vi "Create Link.vi"(8 "Error In":errorcluster, 9 "Remote Link Path":string, 10 "Remote Source Path":string, 11 "SFTP In":refnum<class "SFTP.lvclass">) -> (0 "Error Out":errorcluster, 3 "SFTP Out":refnum<class "SFTP.lvclass">)   [LabVIEW 2018, in "Toolkit.lvlib" / "SFTP.lvclass"]
uses:
  SFTP.lvclass
  SFTP.lvclass/SFTP.ctl
  Session/Session.lvclass/Session.ctl
  SSH/SSH.lvclass/SSH.ctl
  Toolkit.lvlib
  Session/Session.lvclass
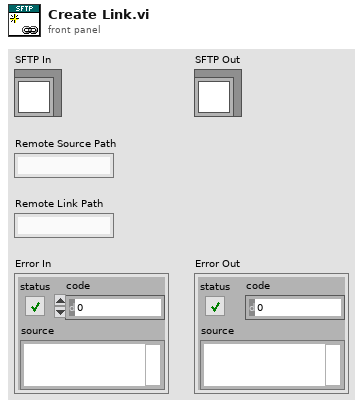
[diagram p1: front panel]
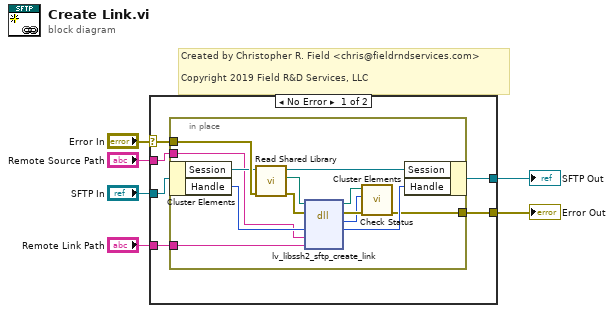
[diagram p0: block diagram]
diagram:
  # "Created by Christopher R. Field <chris@fieldrndservices.com>\n\nCopyright 2019 Field R&D Services, LLC"
  n1 = case shown="No Error" "Error In" {
    selector: "Error In" -> [w12 w27]
    tunnel: [w11 w27] -> w5
    tunnel: "SFTP In" -> [w10 w26]
    tunnel: [w9 w26] -> w3
    tunnel: "Remote Source Path" -> [w8 _]
    tunnel: "Remote Link Path" -> [w7 _]
    frame No Error {
      n2 = in-place {
        in-place-border: w12 -> [w20]
        in-place-border: [w21] -> w11
        in-place-border: w8 -> [w14]
        in-place-border: w7 -> [w13]
        n3 = in-place-cluster #1(w10) -> ("Session"=w19:refnum<class "Session.lvclass">, "Handle"=w15:u64)
        n4 = call "Read Shared Library.vi"("Error In"=w20, "Session In"=w19) -> ("Erorr Out"=w17:errorcluster, "libssh2lv Shared Library"=w16:path, "Session Out"=w18:refnum<class "Session.lvclass">)  [unwired: 7 in]
        n5 = dll-call lib="libssh2lv.*" fn="lv_libssh2_sftp_create_link"(path in=w16, error in=w17, "handle"=w15, "source_path"=w14, "link_path"=w13) -> (path out=w23:path, error out=w24:errorcluster, "status"=w22:i32, "handle"=w25:u64)  [unwired: 3 in]
        n6 = call "Check Status.vi"("Error In"=w24, "Status"=w22, "lv-libssh2 Shared Library In"=w23) -> ("Error Out"=w21:errorcluster)  [unwired: 7 in, 1 out]
        n7 = in-place-cluster #1("Session"=w18, "Handle"=w25) -> (w9:refnum<class "SFTP.lvclass">)
      }
    }
    frame Error {
    }
  }
  "Error Out" <- w5
  "SFTP Out" <- w3
